vi "Write to Hardware.vi"(7 "Valid Triggers":bool, 8 "error in (no error)":errorcluster, 9 "Trigger Values":dbl[](array[numeric]), 10 "Values in":dbl[](array[numeric]), 11 "Tx Scheduled Execution Unit in":refnum<class "Tx Scheduled Labels Execution Unit.lvclass">) -> (0 "error out":errorcluster, 1 "Trigger Values out":dbl[](array[numeric]), 2 "Values out":dbl[](array[numeric]), 3 "Tx Scheduled Execution Unit out":refnum<class "Tx Scheduled Labels Execution Unit.lvclass">)   [LabVIEW 2024, in "AIM ARINC 429 Engine.lvlib" / "Implementation.lvlib" / "Tx Scheduled Labels Execution Unit.lvclass"]
uses:
  Tx Scheduled Labels Execution Unit.lvclass
  C:/dev/niveristand-aim-arinc429-custom-device/Source/Custom Device Support/Engine/Implementation/Execution Unit/Execution Unit.lvclass
  Execution Unit/Execution Unit.lvclass/Execution Unit.ctl
  Tx Scheduled Labels Execution Unit.lvclass/Tx Scheduled Labels Execution Unit.ctl
  Custom Device/Write Error to System Log.vi/ca55ed61-c1f5-4d13-8aef-490b87d2cf89.vi
  <vilib>/NI VeriStand/Custom Device Tools/Custom Device Utility Library/NI VeriStand - Print Debug Line.vi
  Execution Unit/Execution Unit.lvclass
  Hardware API/AIM ARINC 429 Hardware API.lvlib
  Custom Device/Custom Device.lvlib
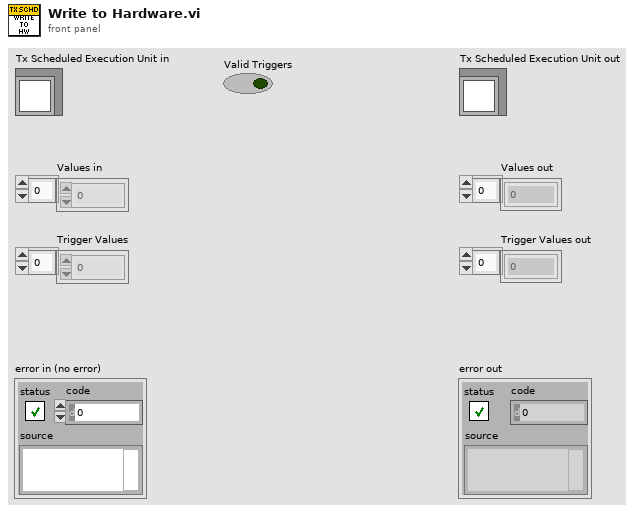
[diagram p1: front panel]
types:
  T1 = typedef "RT Hardware Channel Settings.ctl" = cluster{"channel #":u16, "channel handle":u64, "labels settings for RT":T2[], "speed":T10}
  T2 = typedef "RT Label Settings.ctl" = cluster{"Name":string, "xmlName":string, "label":T3, "transfer period":u32, "SDI_Enabled":bool, "SDI":u8, "parameter driver data":T4, "transfer type":T8, "has timestamp?":bool, "Label Disable/Trigger Channel Reference":T7, "Message Handle":u64, "Initialized?":bool, "Word Initial Raw Value":u32, "Label Timestamp Channel Data Reference":T9, "disabled":bool, "modified":bool}
  T3 = typedef "Label.ctl" = u8
  T4 = typedef "RT Parameters.ctl" = cluster{"parameter definitions":T5[], "Tx parameter refs":T7[]}
  T5 = typedef "Parameter Definition.ctl" = cluster{"start index":i32, "size":i32, "encoding":T6, "signed":bool, "scale multiplier":dbl, "scale offset":dbl, "default value":dbl}
  T6 = typedef "Encoding and Decoding.lvlib/Encoding.ctl" = enum16{"BNR", "BCD", "Discrete"}
  T7 = typedef "Custom Device API.lvlib/Custom Device Item Ref.ctl" = u64
  T8 = typedef "Transfer Type.ctl" = enum16{"Scheduled", "Acyclic", "Block", "Strobe"}
  T9 = typedef "Custom Device API.lvlib/Data Reference.ctl" = i32
  T10 = typedef "Transfer Speed.ctl" = enum16{"LO (12.5 kb/s)", "HI (100 kb/s)"}
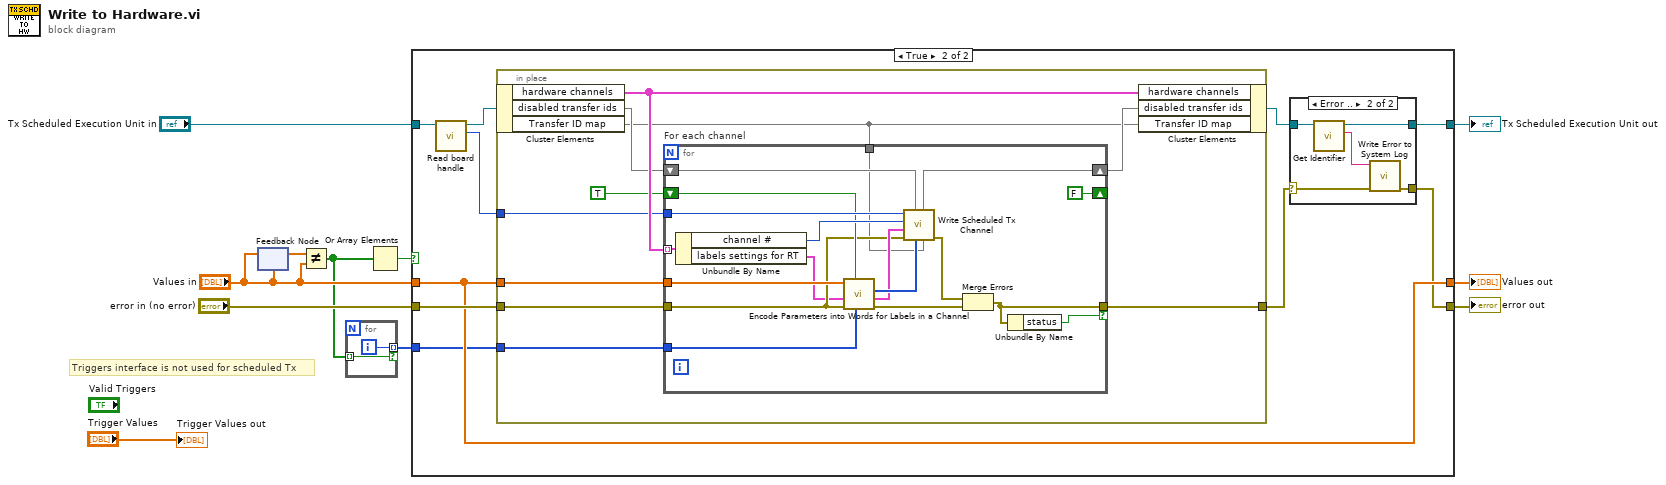
[diagram p0: block diagram]
diagram:
  # "Triggers interface is not used for scheduled Tx"
  n1 = feedback-in #1("Values in") -> ()
  n2 = feedback #1("Values in") -> (w11:dbl[])
  n3 = Not Equal?(x=w11, y="Values in") -> (x != y?=w2:bool[])
  n4 = for {
    tunnel: w2 -> [w12] mode=indexing
    tunnel: [w13] -> w1 mode=indexing if=w12
    i -> [w13]
  }
  n5 = Or Array Elements(Boolean array=w2) -> (logical OR=w3:bool)
  n6 = case shown="True" w3 {
    tunnel: "Values in" -> [w15 w22]
    tunnel: "Tx Scheduled Execution Unit in" -> [w14 w26]
    tunnel: "error in (no error)" -> [w16 w23]
    tunnel: [w16 w18] -> w7
    tunnel: [w15 w22] -> w6
    tunnel: [w14 w20] -> w5
    tunnel: w1 -> [_ w17]
    frame False {
    }
    frame True {
      n7 = call "Read board handle.vi"("Execution Unit in"=w26) -> ("board handle"=w24:u8, "Execution Unit out"=w25:refnum<class "Tx Scheduled Labels Execution Unit.lvclass">)  [unwired: 8 in, 1 out]
      n8 = in-place {
        in-place-border: w24 -> [w42]
        in-place-border: w23 -> [w41]
        in-place-border: w22 -> [w40]
        in-place-border: [w39] -> w19
        in-place-border: w17 -> [w35]
        n9 = in-place-cluster #2(w25) -> ("hardware channels"=w43:T1[], "disabled transfer ids"=w37:set{u32}, "Transfer ID map"=w34:map{u32, u32})
        n10 = for "For each channel" {
          tunnel: w43 -> [w61] mode=indexing
          tunnel: w42 -> [w59]
          shift-right: [FALSE] -> _
          shift-left: TRUE -> [w55]
          tunnel: w40 -> [w58]
          tunnel: w41 -> [w49]
          tunnel: [w51] -> w39 if=w50
          shift-right: [w47] -> w36
          shift-left: w37 -> [w48]
          tunnel: w35 -> [w45]
          tunnel: w34 -> [w44]
          n11 = Unbundle By Name(w61) -> ("channel #"=w60:u16, "labels settings for RT"=w46:T2[])
          n12 = call "Encode Parameters into Words for Labels in a Channel.vi"("modified indices"=w45, "reset index"=w55, "error in (no error)"=w49, "labels settings for RT in"=w46, "Parameter Values in"=w58) -> ("error out"=w52:errorcluster, "labels settings for RT out"=w54:T2[], "data words out"=w57:u32[])  [unwired: 4 in]
          n13 = call "Write Scheduled Tx Channel.vi"("Transfer ID map"=w44, "data in"=w57, "disabled transfers"=w48, "error in"=w49, "labels settings for RT"=w54, "channel number in"=w60, "board handle in"=w59) -> ("error out"=w53:errorcluster, "disabled transfers out"=w47:set{u32})  [unwired: 1 in, 2 out]
          n14 = Merge Errors(w53, w52) -> (w51:errorcluster)
          n15 = Unbundle By Name(w51) -> ("status"=w50:bool)
        }
        n16 = in-place-cluster #2("hardware channels"=w43, "disabled transfer ids"=w36, "Transfer ID map"=w34) -> (w21:refnum<class "Tx Scheduled Labels Execution Unit.lvclass">)
      }
      n17 = case shown="Error .." w19 {
        selector: w19 -> [w27 w30]
        tunnel: w21 -> [w28 w33]
        tunnel: [w28 w32] -> w20
        tunnel: [w27 w29] -> w18
        frame No Error {
        }
        frame Error {
          n18 = call-dynamic "Get Identifier.vi"("Execution Unit Implementation in"=w33) -> ("Identifier"=w31:string, "Execution Unit Implementation out"=w32:refnum<class "Tx Scheduled Labels Execution Unit.lvclass">)  [unwired: 8 in, 1 out]
          n19 = call "Write Error to System Log.vi"("error in"=w30, "identifier"=w31) -> ("error out"=w29:errorcluster)  [unwired: 9 in]
        }
      }
    }
  }
  "error out" <- w7
  "Tx Scheduled Execution Unit out" <- w5
  "Values out" <- w6
  "Trigger Values out" <- "Trigger Values"
